vi "I64_To_U8_Arr.vi"(1 "U64":i64) -> (0 "data":u8[](array[numeric]))   [LabVIEW 2011]
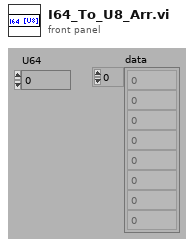
[diagram p1: front panel]
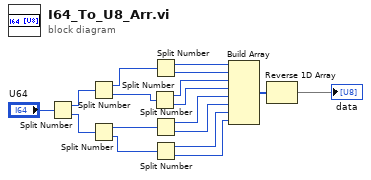
[diagram p0: block diagram]
diagram:
  n1 = Split Number(x="U64") -> (hi(x)=w16:u32, lo(x)=w15:u32)
  n2 = Split Number(x=w16) -> (hi(x)=w13:u16, lo(x)=w14:u16)
  n3 = Split Number(x=w15) -> (hi(x)=w12:u16, lo(x)=w11:u16)
  n4 = Split Number(x=w14) -> (hi(x)=w8:u8, lo(x)=w7:u8)
  n5 = Split Number(x=w13) -> (hi(x)=w10:u8, lo(x)=w9:u8)
  n6 = Split Number(x=w12) -> (hi(x)=w6:u8, lo(x)=w5:u8)
  n7 = Split Number(x=w11) -> (hi(x)=w4:u8, lo(x)=w3:u8)
  n8 = Build Array(w10, w9, w8, w7, w6, w5, w4, w3) -> (w2:u8[])
  n9 = Reverse 1D Array(array=w2) -> (reversed array=→"data":u8[])
